vi "Host.vi"() -> ()   [LabVIEW 2025]
uses:
  <vilib>/FPGAPlugInAG/cRIO-9035/niLvFpga_Open_cRIO-9035.vi
  <vilib>/rvi/interface/common/dynamic/niFpgaDynamicAddResources.vi
  <vilib>/FPGAPlugInAG/Dynamic/niLvFpga_Reset_Dynamic.vi
  <vilib>/Utility/error.llb/Error Cluster From Error Code.vi
  <vilib>/rvi/errors/niLvFpgaAdjustHostInterfaceError.vi
  <vilib>/FPGAPlugInAG/Dynamic/niLvFpga_Run_Dynamic.vi
  <vilib>/FPGAPlugInAG/Dynamic/niLvFpga_Close_Dynamic.vi
  <vilib>/rvi/interface/nirviOpenFPGA/nirviOpenFPGA.xnode
  FPGA Bitfiles/hmmlponfpgav3_FPGATarget_Target_NQ204g-iF-I.lvbitx
  Target.vi
  <vilib>/rvi/interface/nirviMethod/nirviMethod.xnode
  <vilib>/rvi/interface/nirviCloseFPGA/nirviCloseFPGA.xnode
  <vilib>/rvi/errors/niLvFpgaMergeErrorWithErrorCode.vi
  <vilib>/FPGAPlugInAG/Dynamic/niLvFpga_ReadFifo_Dynamic.vi
  <vilib>/FPGAPlugInAG/Dynamic/niLvFpga_WriteFifo_Dynamic.vi
panel:
  out "Unhealthy%":sgl[](array[numeric])
  out "Window(s)":dbl[][](array[numeric])
  out "input":dbl[][](array[numeric])
  out "Healthy%":sgl[](array[numeric])
  out "Window":sgl[](graph)
  out "size(s) 2":i32
  out "output array":sgl[](array[numeric])
  out "size(s)":i32[](array[numeric])
  out "Uncontrolled Acceleration":dynamicdata(graph)
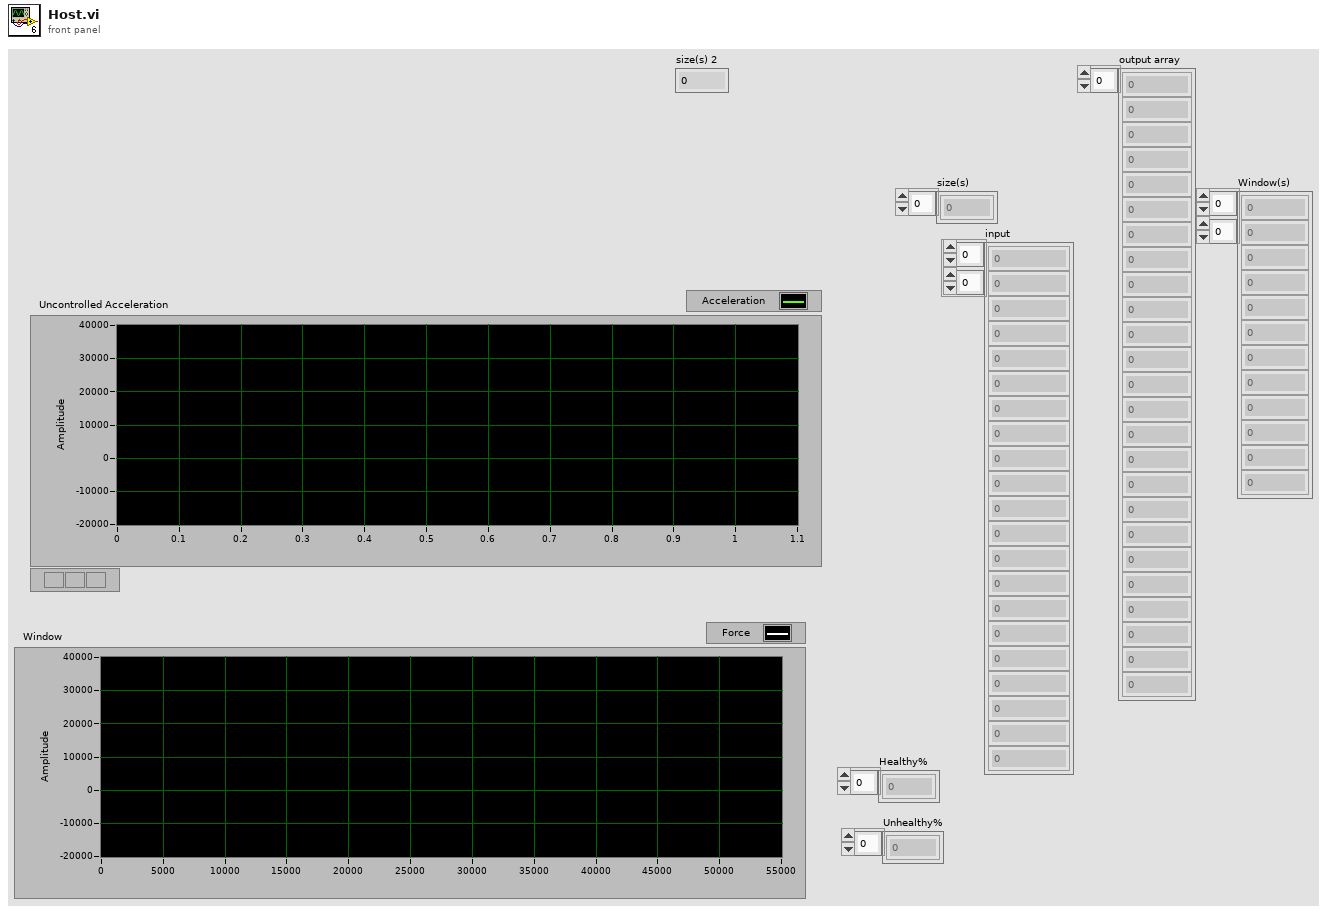
[diagram p1: front panel]
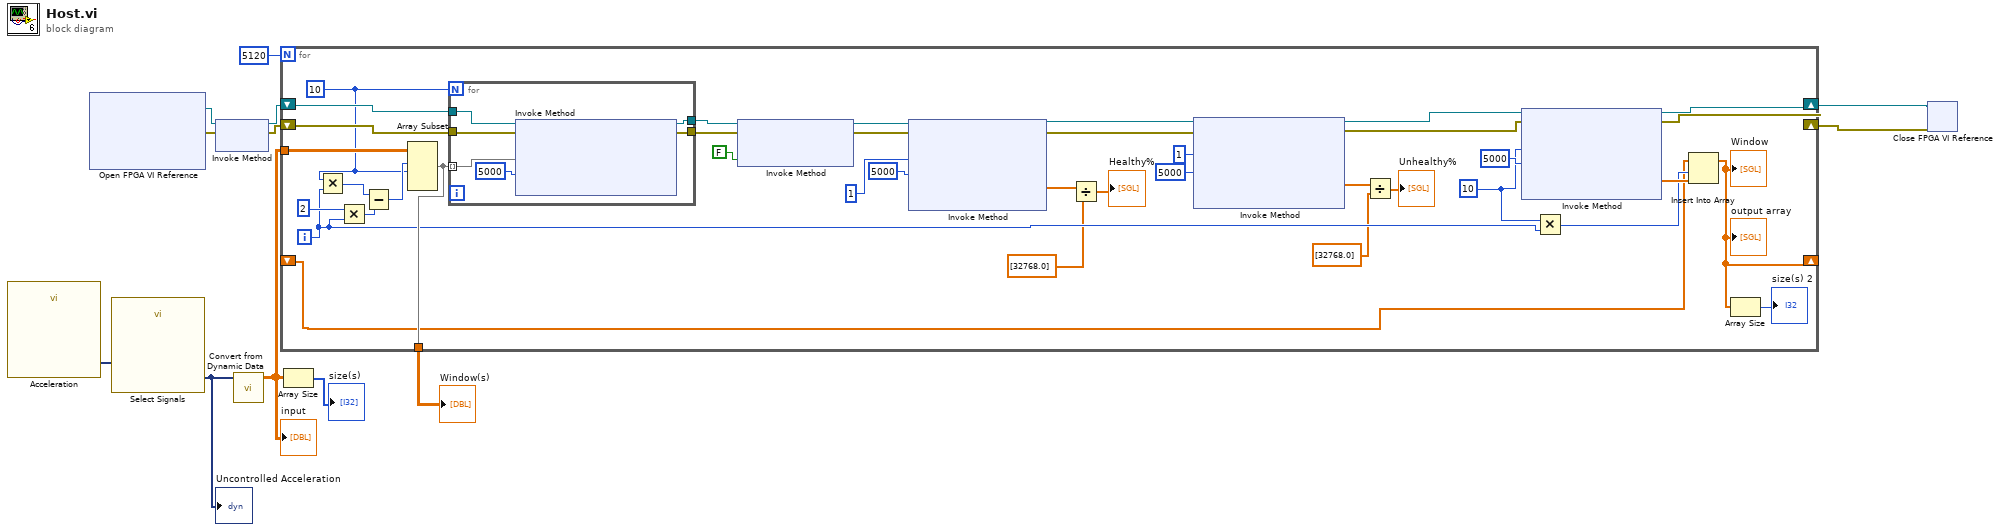
[diagram p0: block diagram]
diagram:
  n1 = call "Acceleration"() -> ("Signals"=w12:dynamicdata)  [unwired: 6 in, 5 out]
  n2 = xnode "Open FPGA VI Reference"() -> ("FPGA VI Reference Out"=w11:refnum<k20>, "error out"=w8:errorcluster)  [unwired: 2 in]
  n3 = call "Select Signals"("Signals"=w12) -> ("Signal Out"=w7:dynamicdata)  [unwired: 9 in, 1 out]
  "Uncontrolled Acceleration" <- w7
  n4 = xnode "Invoke Method"("FPGA VI Reference In"=w11, "error in"=w8) -> ("FPGA VI Reference Out"=w10:refnum<k20>, "error out"=w9:errorcluster)
  n5 = call "Convert from Dynamic Data"("Dynamic Data Type"=w7) -> ("Array"=w2:dbl[][])  [unwired: 3 in]
  "input" <- w2
  n6 = for {
    N: 5120 -> [_]
    shift-right: [w29] -> w5
    shift-left: w10 -> [w50]
    shift-right: [w34] -> w4
    shift-left: w9 -> [w49]
    tunnel: w2 -> [w41]
    tunnel: [w40] -> w1
    shift-right: [w33] -> _
    shift-left: _ -> [w30]
    i -> [w27]
    w31 = u32 10 ("Number of Elements")
    w25 = 10
    n7 = Multiply(x=w25, y=w27) -> (x*y=w39:i32)
    n8 = Multiply(x=2 ("y"), y=w27) -> (x*y=w26:i32)
    n9 = Subtract(x=w39, y=w26) -> (x-y=w38:i32)
    n10 = Array Subset(array=w41, index (row)=w38, length (row)=w25) -> (w40:dbl[][])  [unwired: 2 in]
    n11 = for {
      N: w25 -> [_]
      tunnel: w50 -> [w56]
      tunnel: w49 -> [w55]
      tunnel: [w53] -> w45
      tunnel: [w52] -> w44
      tunnel: w40 -> [w51] mode=indexing
      n12 = xnode "Invoke Method"("FPGA VI Reference In"=w56, "error in"=w55, "Data"=w51, "Timeout (ms)"=5000) -> ("FPGA VI Reference Out"=w53:refnum<k20>, "error out"=w52:errorcluster)  [unwired: 1 out]
    }
    n13 = xnode "Invoke Method"("FPGA VI Reference In"=w45, "error in"=w44, "Wait Until Done (F)"=FALSE) -> ("FPGA VI Reference Out"=w47:refnum<k20>, "error out"=w46:errorcluster)
    n14 = xnode "Invoke Method"("FPGA VI Reference In"=w47, "error in"=w46, "Number of Elements"=u32 1, "Timeout (ms)"=5000) -> ("FPGA VI Reference Out"=w24:refnum<k20>, "error out"=w23:errorcluster, "Data"=w17:sgl[])  [unwired: 1 out]
    n15 = Divide(x=w17, y=sgl[] [32768.0]) -> (x/y=→"Healthy%":sgl[])
    n16 = xnode "Invoke Method"("FPGA VI Reference In"=w24, "error in"=w23, "Number of Elements"=u32 1, "Timeout (ms)"=5000) -> ("FPGA VI Reference Out"=w21:refnum<k20>, "error out"=w22:errorcluster, "Data"=w14:sgl[])  [unwired: 1 out]
    n17 = Divide(x=w14, y=sgl[] [32768.0]) -> (x/y=→"Unhealthy%":sgl[])
    n18 = xnode "Invoke Method"("FPGA VI Reference In"=w21, "error in"=w22, "Number of Elements"=w31, "Timeout (ms)"=5000) -> ("FPGA VI Reference Out"=w29:refnum<k20>, "error out"=w34:errorcluster, "Data"=w36:sgl[])  [unwired: 1 out]
    n19 = Multiply(x=w31, y=w27) -> (x*y=w35:u32)
    n20 = Insert Into Array(array=w30, index=w35, new element=w36) -> (w33:sgl[])
    "Window" <- w33
    "output array" <- w33
    n21 = Array Size(array=w33) -> (size(s)=→"size(s) 2":i32)
  }
  "Window(s)" <- w1
  n22 = Array Size(array=w2) -> (size(s)=→"size(s)":i32[])
  n23 = xnode "Close FPGA VI Reference"("FPGA VI Reference In"=w5, "error in"=w4) -> ()  [unwired: 1 out]
